vi "Detect Tester.vi"(8 "error in":errorcluster) -> (0 "error out":errorcluster, 3 "Tester Detected":bool)   [LabVIEW 2024, in "RT Management.lvlib"]
uses:
  RT Management.lvlib
  ECU Internal Communications/Notifiers - Get.vi
  ECU Internal Communications/ECU InterComm.lvlib
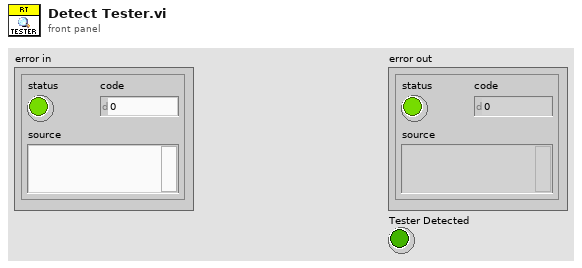
[diagram p1: front panel]
types:
  T1 = typedef "ECU InterComm.lvlib/ECU Notifiers.ctl" = cluster{"Tester Detected":refnum<notifier>, "ECU Released":refnum<notifier>}
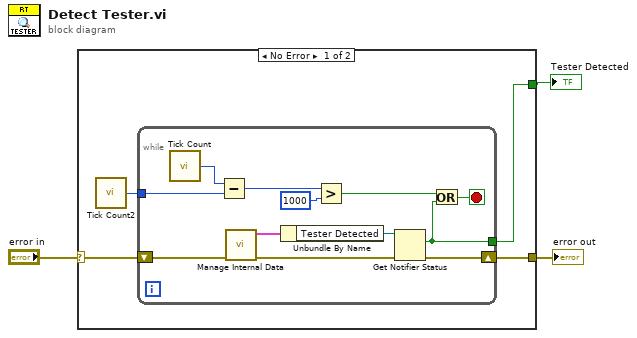
[diagram p0: block diagram]
diagram:
  n1 = case shown="No Error" "error in" {
    selector: "error in" -> [w6 w20]
    tunnel: [w5 w20] -> w3
    tunnel: [w4 _] -> w1
    frame No Error {
      n2 = call "Tick Count2"() -> ("Tick Count(mSec)"=w7:u32)
      n3 = while {
        shift-right: [w8] -> w5
        shift-left: w6 -> [w9]
        tunnel: w7 -> [w18]
        tunnel: [w13] -> w4
        stop <- w14 stop-if-true
        n4 = call "Tick Count"() -> ("Tick Count(mSec)"=w19:u32)
        n5 = Subtract(x=w19, y=w18) -> (x-y=w16:u32)
        n6 = call-poly "Manage Internal Data.vi"("error in"=w9) -> ("error out"=w10:errorcluster, "ECU Notifiers"=w12:T1)  [unwired: 9 in]
        n7 = Unbundle By Name(w12) -> ("Tester Detected"=w11:refnum<notifier>)
        n8 = Greater?(x=w16, y=u32 1000) -> (0:w15:bool)
        n9 = Get Notifier Status(notifier=w11, error in (no error)=w10) -> (current notification=w13:bool, error out=w8:errorcluster)  [unwired: 3 out]
        n10 = Or(x=w15, y=w13) -> (x .or. y?=w14:bool)
      }
    }
    frame Error {
    }
  }
  "error out" <- w3
  "Tester Detected" <- w1
